vi "DHE_DRV_get_expose_status.vi"(11 "error in (no error)":errorcluster) -> (6 "sequence stoped":bool, 8 "coadd stoped":bool, 15 "error out":errorcluster)   [LabVIEW 2016]
doc: "This VI closes the I/O interface with the instrument."
uses:
  c/lib/libarcDHE.so
panel:
  in  "coadd":i32
  in  "sequence":i32
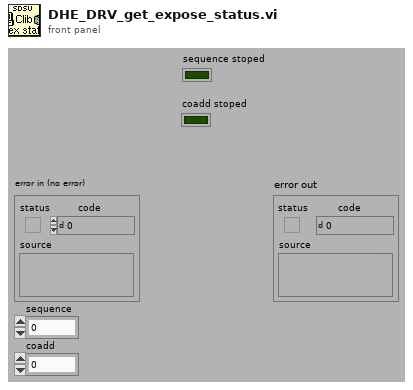
[diagram p1: front panel]
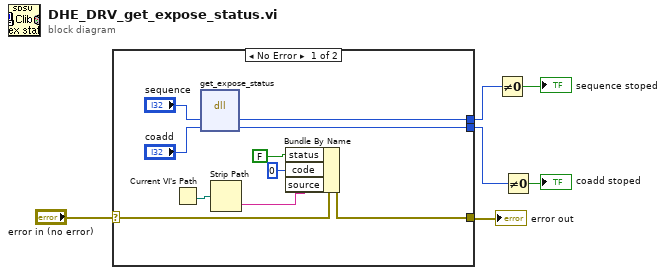
[diagram p0: block diagram]
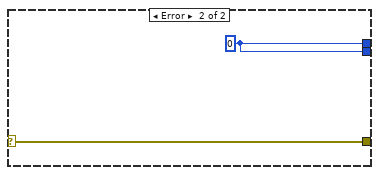
[diagram p2: hidden frame]
diagram:
  n1 = case shown="No Error" "error in (no error)" {
    selector: "error in (no error)" -> [w13 w18]
    tunnel: [w14 w18] -> w6
    tunnel: [w10 w17] -> w4
    tunnel: [w9 w17] -> w1
    frame No Error {
      n2 = Current VI's Path() -> (path=w16:path)
      n3 = dll-call lib="home/simager/panview/PAN/Modules/SDSU/private/c/lib/libarcDHE.so" fn="get_expose_status"("sequence"="sequence", "coadd"="coadd") -> ("sequence"=w10:i32, "coadd"=w9:i32)  [unwired: 3 in, 3 out]
      n4 = Strip Path(path=w16) -> (name=w15:string)  [unwired: 1 out]
      n5 = Bundle By Name(cluster=w13, "status"=FALSE, "code"=0, "source"=w15) -> (w14:errorcluster)
    }
    frame Error {
      w17 = 0 ("sequence")
    }
  }
  "error out" <- w6
  n6 = Not Equal To 0?(x=w4) -> (x != 0?=→"sequence stoped":bool)
  n7 = Not Equal To 0?(x=w1) -> (x != 0?=→"coadd stoped":bool)
